vi "SwissSPAD Live_Decode SS3 FPGA Data_DVI.vi"(8 "Error In":errorcluster, 9 "Buffer Size (# 8-bit Images)":i32, 10 "SwissSPAD Live Internal Variables":T1={"okCFrontPanelDevices Refnum"=refnum, "Bottom Device Refnum"=refnum, "Display Image"=refnum, "# Live Images"=0, "relative s"=0.0, "# Image Sets"=0, "Message"="", "Current Image Set"=0, "# Datasets in Series"=0, "Current Dataset"=0, "Live Mode"=FALSE, "Recording Mode"=FALSE, "Record Button"=refnum, "\nLive Button"=refnum, "SwissSPAD Live Gate Image Data Q Name"="SS2 Live Gate Data Q", "Discard First Image"=FALSE, "Image Information"={"Save ROI Only"=FALSE, "Left"=0, "Top"=0, "Right"=0, "Bottom"=0, "Use Current ROI"=FALSE}, "Image Binning Options"={"Use Image Binning"=FALSE, "X Bin"=1, "Y Bin"=1}, "Bottom FPGA Serial Number"="", "Detector PCB Version"=enum."SS2 PCB1", "# Acquisitions"=1, "10 bits"=FALSE, "Top FPGA Serial Number"="", "Top Device Refnum"=refnum, "okCFrontPanel Refnum"=refnum} {"# Acquisitions" min=1; "Image Binning Options"."Y Bin" min=1; "Image Binning Options"."X Bin" min=1}) -> ()   [LabVIEW 2021]
uses:
  SwissSPAD Live_Internal Variables.ctl
  D:/UCLA Thinkpad Google Drive/LabVIEW 2021 SP1/builds/SwissSPAD Live Distribution/Opal Kelly/C# Wrapper/v5.0.2/libFrontPanel-csharp.dll
  Opal Kelly/C# Wrapper/v5.0.2/libFrontPanel-csharp.dll
  <vilib>/vision/Image Controls.llb/IMAQ Image.ctl
  SwissSPAD Live_Image ROI Information.ctl
  Phasor/Image Binning Options.ctl
  SwissSPAD Live_SSx PCB Version.ctl
  SwissSPAD Live_Settings List.ctl
  SwissSPAD Live_SS3 Displayed Image v2.ctl
  LV Tools/Logical Processors Used.vi
  Time/High Resolution Timing.vi
  <vilib>/vision/NI_Vision_Development_Module.lvlib
  Notebook/Notebook.lvlib
  Rich Text Box/Rich Text Box.lvlib
  Variant/Variant to Data/Variant to Data.lvlib
panel:
  out "# 8-bit image pairs queued":i32
  out "Activate Trigger Error Out":errorcluster
  out "8-bit Image Count":i32
  out "Error Out":errorcluster
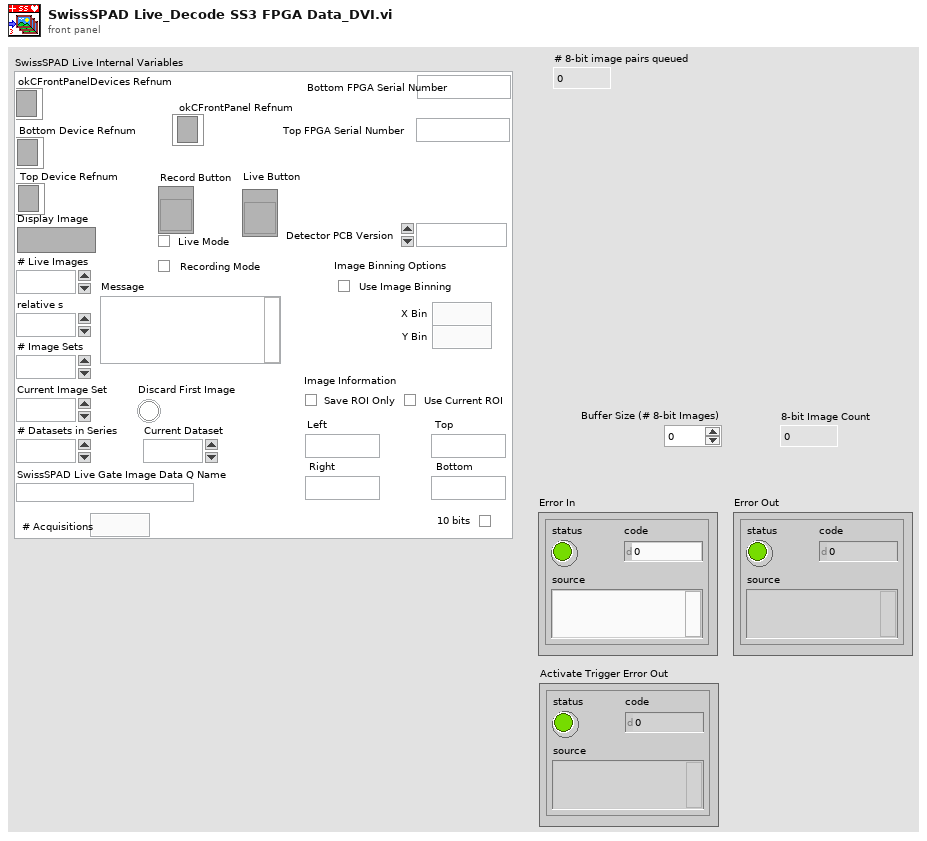
[diagram p1: front panel]
types:
  T1 = typedef "SwissSPAD Live_Internal Variables.ctl" = cluster{"okCFrontPanelDevices Refnum":refnum<k24>, "Bottom Device Refnum":refnum<k24>, "Display Image":T2, "# Live Images":i32, "relative s":dbl, "# Image Sets":i32, "Message":string, "Current Image Set":i32, "# Datasets in Series":i32, "Current Dataset":i32, "Live Mode":bool, "Recording Mode":bool, "Record Button":refnum<vi>, "\nLive Button":refnum<vi>, "SwissSPAD Live Gate Image Data Q Name":string, "Discard First Image":bool, "Image Information":T3, "Image Binning Options":T4, "Bottom FPGA Serial Number":string, "Detector PCB Version":T5, "# Acquisitions":u32, "10 bits":bool, "Top FPGA Serial Number":string, "Top Device Refnum":refnum<k24>, "okCFrontPanel Refnum":refnum<k24>}
  T2 = typedef "IMAQ Image.ctl" = refnum<image>
  T3 = typedef "SwissSPAD Live_Image ROI Information.ctl" = cluster{"Save ROI Only":bool, "Left":u16, "Top":u16, "Right":u16, "Bottom":u16, "Use Current ROI":bool}
  T4 = typedef "Image Binning Options.ctl" = cluster{"Use Image Binning":bool, "X Bin":i32, "Y Bin":i32}
  T5 = typedef "SwissSPAD Live_SSx PCB Version.ctl" = enum16{"unknown", "SS2 PCB1", "SS2 PCB2", "SS3 PCB1"}
  T6 = typedef "SwissSPAD Live_Settings List.ctl" = enum16{"FPGA:Bottom Half", "FPGA:Top Half", "FPGA:Bottom Bitfile Path", "FPGA:Top Bitfile Path", "FPGA:Bottom Bitstream Version", "FPGA:Top Bitstream Version", "FPGA:Auto Reset FPGA", "FPGA:Bottom FPGA Serial Number", "FPGA:Top FPGA Serial Number", "FPGA:Detector PCB Version", "Acquisition Parameters:Microlens", "Acquisition Parameters:SS2 DAQ Parameters", "Acquisition Parameters:Gate Configuration Array", "Acquisition Parameters:SS3 DAQ Parameters", "Acquisition Parameters:Buffer Size (# 8-bit Gates)", "File Information:File Information", "File Information:# Datasets in Series", "File Information:Scrambled File Flag", "File Information:SS3 Gate Slip Correction", "File Information:SS3 Hot Pixel Mismatch Detection", "File Information:Delay between Datasets", "File Information:Save Sum of All Gates Preview", "Image Parameters:Image ROI Information", "Image Parameters:Image Binning Options", "Image Parameters:SS3 Displayed Image", "Image Parameters:Image Display Options", "Image Parameters:Use Histogram Cursors", "Image Parameter:FPGA Data to Display", "UI Settings:Histogram Bins Number", "UI Settings:Histogram Bin Size", "UI Settings:Use Image Display Options", "UI Settings:Verbose Settings", "UI Settings:Verbose Saving"}
  T7 = typedef "SwissSPAD Live_SS3 Displayed Image v2.ctl" = enum16{"G2 Gate", "INT Gate", "INT - G2"}
  T8 = typedef "Image Type" = u32
  T9 = typedef "Rich Text Box.lvlib/Text Formatting.ctl" = cluster{"Font":string, "Text Color":T10, "Text Background Color":T10, "Text Style":enum16{"Regular", "Bold", "Italic", "Underline", "Strikeout"}, "Font Size (Points)":dbl, "Text Alignment":i32}
  T10 = typedef "Rich Text Box.lvlib/Text Colors.ctl" = enum16{"Unchanged", "Black", "Blue", "Brown", "Gray", "Green", "Orange", "Pink", "Red", "White"}
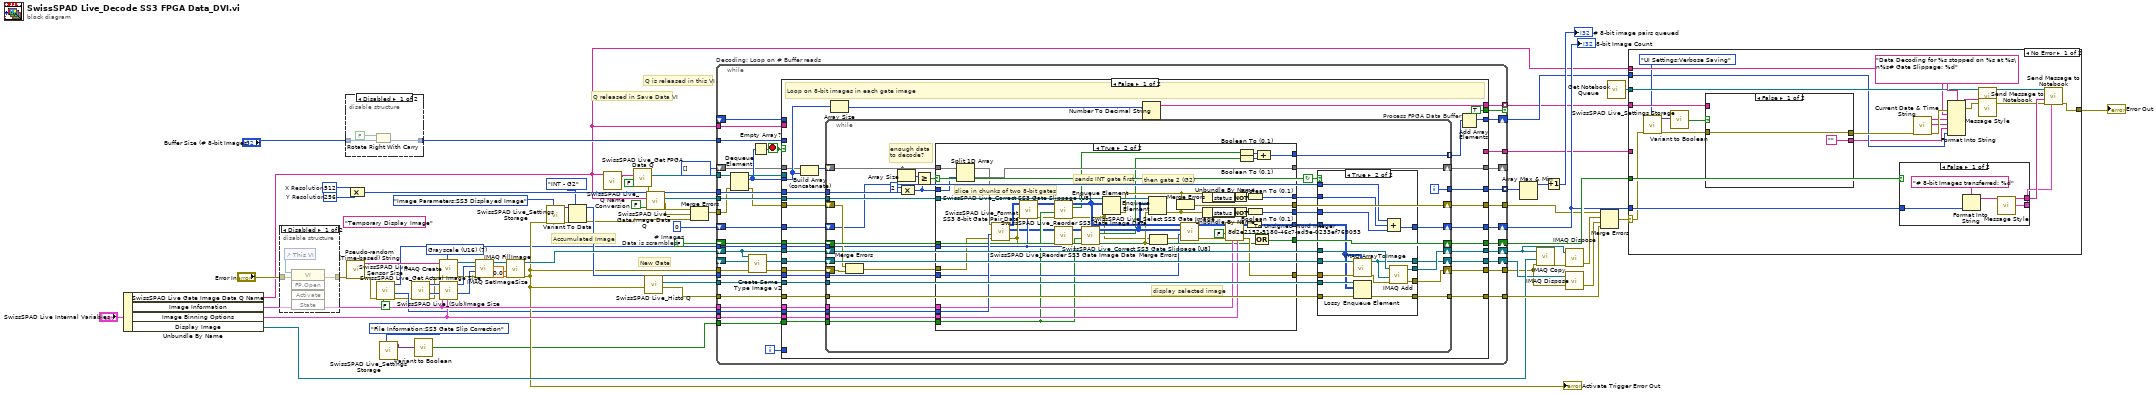
[diagram p0: block diagram]
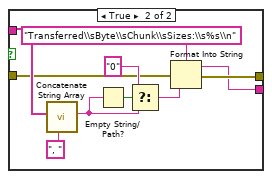
[diagram p3: hidden frame]
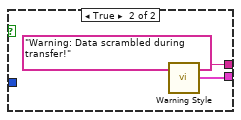
[diagram p4: hidden frame]
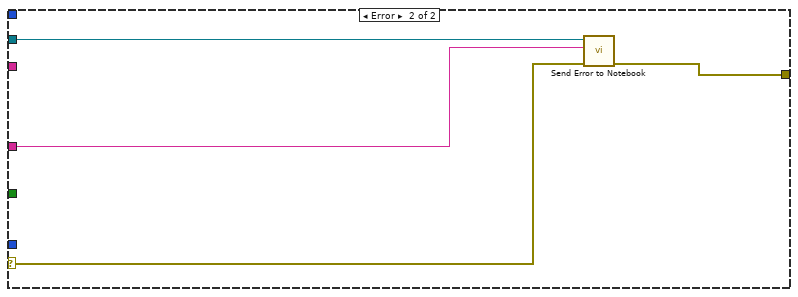
[diagram p5: hidden frame]
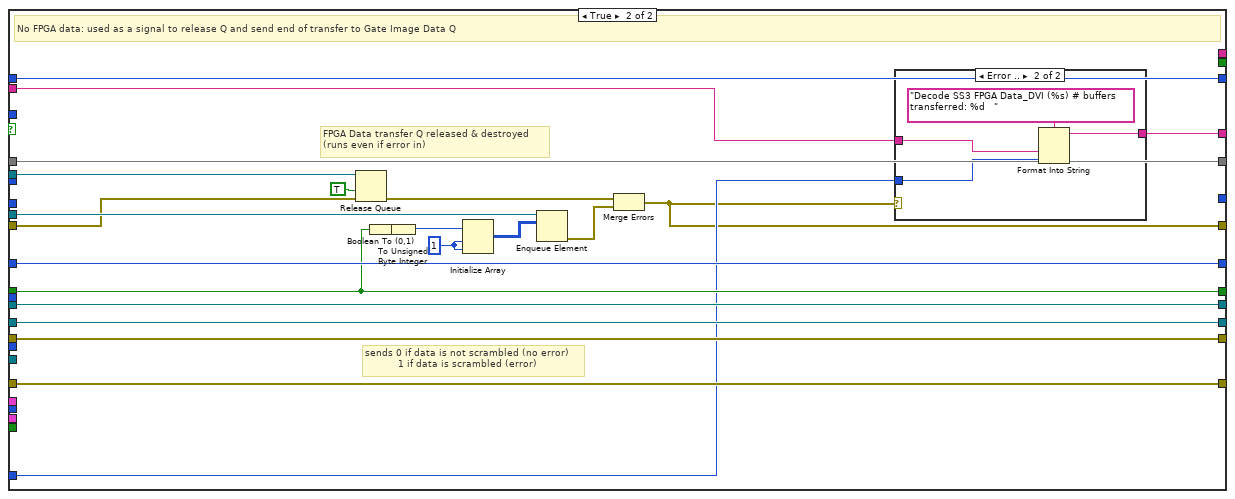
[diagram p8: hidden frame]
diagram:
  w56 = FALSE  # Data is scrambled
  w59 = T8 7 items=["Grayscale (U8)", "Grayscale (I16)", "Grayscale (SGL)", "Complex (CSG)", "RGB (U32)", "HSL (U32)", "RGB (U64)", "Grayscale (U16)"] ("Image Type")
  (unwired) "Temporary Display Image" ("Image Name")
  w68 = 0  # # Images
  w43 = 256  # Y Resolution
  w72 = 512  # X Resolution
  # "New Gate"
  # "Accumulated Image"
  # "Q released in Save Data VI"
  # "Q is released in this VI"
  n1 = Unbundle By Name("SwissSPAD Live Internal Variables") -> ("SwissSPAD Live Gate Image Data Q Name"=w8:string, "Image Information"=w55:T3, "Image Binning Options"=w54:T4, "Display Image"=w52:T2)
  n2 = disable-structure shown="Disabled" {
    disable-tunnel: "Error In" -> [w74 w76]
    disable-tunnel: [w73 w76] -> w35
    frame Disabled {
      n3 = control-ref of="This VI"() -> (w75:refnum<vi>)
      n4 = invoke class="VI" method="FP.Open"(reference=w75, error in=w74) -> (error out=w73:errorcluster)  [unwired: 3 in, 4 out]
    }
    frame Enabled {
    }
  }
  n5 = disable-structure shown="Disabled" {
    disable-tunnel: [w79 w80] -> w39
    disable-tunnel: "Buffer Size (# 8-bit Images)" -> [w78 w80]
    frame Disabled {
      n6 = Rotate Right With Carry(2:w78, 3:FALSE ("carry")) -> (0:w79:i32)  [unwired: 1 out]
    }
    frame Enabled {
      # "Divide by 2 to obtain # INT+G2 pairs"
    }
  }
  n7 = call "Pseudo-random (Time-based) String.vi"("Error In"=w35) -> ("Error Out"=w10:errorcluster, "result string"=w47:string)  [unwired: 9 in]
  n8 = Compound Arithmetic op=MULTIPLY(w72, w43) -> (w58:i32)
  n9 = call "SwissSPAD Live_Sensor Size.vi"("Set/Get(F)"=FALSE, "Error In"=w10) -> ("Error Out"=w14:errorcluster, "Y size"=w16:i32, "X size"=w17:i32)  [unwired: 7 in]
  n10 = call "SwissSPAD Live_Settings Storage.vi"("Settings List"=SwissSPAD_Live_Settings_List."File Information:SS3 Gate Slip Correction") -> ("Variant Data out"=w4:variant)  [unwired: 9 in, 1 out]
  n11 = call "SwissSPAD Live_Get Actual Image Size.vi"("error in (no error)"=w14) -> ("error out"=w11:errorcluster, "Y size"=w12:i32, "X size"=w13:i32)  [unwired: 8 in]
  n12 = call "Variant to Boolean.vi"("Variant"=w4) -> ("Value"=w18:bool)  [unwired: 8 in]
  n13 = call "IMAQ Create"("Image Name"=w47, "Image Type"=w59, "error in (no error)"=w11) -> ("New Image"=w64:T2, "error out"=w65:errorcluster)  [unwired: 2 in]
  n14 = call "SwissSPAD Live_(Sub)Image Size.vi"("Image Binning Options"=w54, "Image Information"=w55, "# Pixel Y in"=w12, "# Pixel X in"=w13) -> ("# Pixel Y out"=w66:i32, "# Pixel X out"=w67:i32)  [unwired: 6 in]
  n15 = call "IMAQ SetImageSize"("error in (no error)"=w65, "Y Resolution"=w66, "X Resolution"=w67, "Image"=w64) -> ("error out"=w62:errorcluster, "Image Out"=w63:T2)  [unwired: 1 in]
  n16 = call "IMAQ FillImage"("error in (no error)"=w62, "Pixel Value (U8, U16, I16, Float)"=sgl 0.0, "Image"=w63) -> ("error out"=w19:errorcluster, "Image Out"=w61:T2)  [unwired: 7 in]
  "Activate Trigger Error Out" <- w19
  n17 = call "SwissSPAD Live_Settings Storage.vi"("Settings List"=SwissSPAD_Live_Settings_List."Image Parameters:SS3 Displayed Image", "Error In"=w19) -> ("Error Out"=w46:errorcluster, "Variant Data out"=w3:variant)  [unwired: 8 in]
  n18 = Variant To Data(error in=w46, type=SwissSPAD_Live_SS3_Displayed_Image_v2."INT - G2" ("Image to Display"), Variant=w3) -> (data=w44:T7, error out=w7:errorcluster)
  n19 = call "SwissSPAD Live_Q Name Conversion.vi"("SwissSPAD Live Gate Data Decode Q Name"=w8) -> ("FPGA Q Name"=w28:string)  [unwired: 10 in]
  n20 = call "SwissSPAD Live_Get FPGA Data Q.vi"("create if not found? (T)"=FALSE, "FPGA Data Q Name"=w28) -> ("error out"=w22:errorcluster, "FPGA Data Q"=w32:refnum<queue>)  [unwired: 8 in]
  n21 = call "SwissSPAD Live_Histo Q.vi"("error in (no error)"=w19) -> ("error out"=w70:errorcluster, "SS2 Live Histo Q"=w71:refnum<queue>)  [unwired: 5 in]
  n22 = call "SwissSPAD Live_Gate Image Data Q.vi"("create if not found? (T)"=FALSE, "SwissSPAD Live Gate Image Data Q Name"=w8) -> ("error out"=w21:errorcluster, "SwissSPAD Live Gate Image Data Q"=w31:refnum<queue>)  [unwired: 7 in, 1 out]
  n23 = Merge Errors(w22, w21, w7) -> (w23:errorcluster)
  n24 = while "Decoding: Loop on # Buffer reads" {
    tunnel: w16 -> [w121]
    tunnel: w19 -> [w114]
    tunnel: w39 -> [w120]
    tunnel: w58 -> [w119]
    shift-right: [w105] -> w26
    shift-left: _ -> [w117]
    tunnel: [w118] -> w25
    tunnel: w23 -> [w103]
    tunnel: [w111] -> w34
    tunnel: w71 -> [w110]
    tunnel: w70 -> [w109]
    tunnel: [w108] -> w69
    shift-right: [w107] -> w50
    shift-left: w61 -> [w116]
    tunnel: w32 -> [w104]
    shift-right: [w113] -> w37
    shift-left: w68 -> [w100]
    tunnel: w55 -> [w99]
    tunnel: w54 -> [w98]
    shift-right: [w97] -> w57
    shift-left: w56 -> [w96]
    tunnel: w17 -> [w94]
    tunnel: w44 -> [w93]
    tunnel: [w92] -> w42 mode=indexing
    tunnel: w31 -> [w112]
    tunnel: [w90] -> w27
    tunnel: w8 -> [w89]
    tunnel: [w88] -> w1 mode=indexing if=w83
    tunnel: w18 -> [w87]
    shift-right: [w85] -> w9
    shift-left: _ -> [w84]
    shift-right: [w81] -> _
    shift-left: u8[] [] -> [w82]
    i -> [w91]
    stop <- w101 stop-if-true
    n25 = Dequeue Element(queue=w104, error in (no error)=w103) -> (queue out=w95:refnum<queue>, element=w86:u8[], error out=w102:errorcluster)  [unwired: 1 in, 1 out]
    n26 = call "Create Same Type Image v2.vi"("error in (no error)"=w114, "Image Dst"=w117, "Image Src"=w116) -> ("error out"=w115:errorcluster, "Image Dst"=w106:T2)  [unwired: 6 in, 1 out]
    n27 = Empty Array?(array=w86) -> (empty?=w101:bool)
    n28 = case shown="False" w101 {
      tunnel: w121 -> [w154 _]
      tunnel: w120 -> [_ _]
      tunnel: w119 -> [w153 _]
      tunnel: [w152 w280] -> w118
      tunnel: w116 -> [w151 w282]
      tunnel: w115 -> [w150 w280]
      tunnel: [w138 w283] -> w113
      tunnel: w112 -> [w149 w278]
      tunnel: [w148 w267] -> w111
      tunnel: w110 -> [w147 _]
      tunnel: w109 -> [w146 w279]
      tunnel: [w145 w279] -> w108
      tunnel: [w144 w282] -> w107
      tunnel: w106 -> [w143 w281]
      tunnel: [w142 w281] -> w105
      tunnel: w102 -> [w141 w268]
      tunnel: w86 -> [w131 _]
      tunnel: w100 -> [w139 w283]
      tunnel: w99 -> [w140 _]
      tunnel: w98 -> [w137 _]
      tunnel: [w135 w277] -> w97
      tunnel: w96 -> [w136 w277]
      tunnel: w95 -> [_ w272]
      tunnel: w94 -> [w134 _]
      tunnel: w93 -> [w133 _]
      tunnel: [w132 _] -> w92
      tunnel: w91 -> [_ w270]
      tunnel: [_ w265] -> w90
      tunnel: w89 -> [_ w264]
      tunnel: [w129 _] -> w88
      tunnel: w87 -> [w128 _]
      tunnel: [w126 w263] -> w85
      tunnel: w84 -> [_ w263]
      tunnel: [TRUE _] -> w83
      tunnel: w82 -> [w123 w262]
      tunnel: [w122 w262] -> w81
      frame False {
        # "Loop on 8-bit images in each gate image"
        n29 = Build Array (concatenate)(w123, w131) -> (w124:u8[])
        n30 = while "Process FPGA Data Buffer" {
          tunnel: w154 -> [w190]
          shift-right: [w184] -> w152
          shift-left: w150 -> [w189]
          shift-right: [w183] -> w122
          shift-left: w124 -> [w188]
          tunnel: w153 -> [w187]
          shift-right: [w165] -> w148
          shift-left: w141 -> [w170]
          tunnel: w147 -> [w182]
          tunnel: w146 -> [w181]
          tunnel: [w180] -> w145
          shift-right: [w179] -> w144
          shift-left: w151 -> [w185]
          shift-right: [w178] -> w142
          shift-left: w143 -> [w186]
          tunnel: w140 -> [w175]
          shift-right: [w176] -> w138
          shift-left: w139 -> [w159]
          tunnel: w137 -> [w174]
          shift-right: [w172] -> w135
          shift-left: w136 -> [w173]
          tunnel: w134 -> [w167]
          tunnel: w133 -> [w166]
          tunnel: [w169] -> w132
          tunnel: w149 -> [w171]
          tunnel: w128 -> [w162]
          tunnel: [w161] -> w127 mode=indexing
          i -> [w169]
          stop <- w158 continue-if-true
          # "enough data to decode?"
          n31 = Merge Errors(w170, w189) -> (w160:errorcluster)
          n32 = Array Size(array=w188) -> (size(s)=w156:i32)
          n33 = Compound Arithmetic op=MULTIPLY(2 ("value"), w187) -> (w155:i32)
          n34 = Greater Or Equal?(x=w156, y=w155) -> (x >= y?=w158:bool)
          n35 = case shown="True" w158 {
            tunnel: w190 -> [_ w241]
            tunnel: [w193 w240] -> w183
            tunnel: [w192 w239] -> w177
            tunnel: w175 -> [_ w238]
            tunnel: w174 -> [_ w237]
            tunnel: w173 -> [w191 w236]
            tunnel: [w191 w235] -> w172
            tunnel: w171 -> [_ w234]
            tunnel: [_ w233] -> w168
            tunnel: w167 -> [_ w232]
            tunnel: w166 -> [_ w231]
            tunnel: [w192 w230] -> w165
            tunnel: [_ w229] -> w164
            tunnel: [_ w228] -> w163
            tunnel: w162 -> [_ w227]
            tunnel: [_ w226] -> w161
            tunnel: w160 -> [w192 w220]
            tunnel: w188 -> [w193 w195]
            tunnel: w155 -> [_ w194]
            frame False {
            }
            frame True {
              # "slice in chunks of two 8-bit gates"
              # "display selected image"
              # "then gate 2 (G2)"
              # "sends INT gate first"
              n36 = Split 1D Array(array=w195, index=w194) -> (first subarray=w225:u8[], second subarray=w240:u8[])
              n37 = call "SwissSPAD Live_Format SS3 8-bit Gate Pair Data.vi"("Error In"=w220, "Y Resolution (250)"=w241, "Flattened Image (512x256x2)"=w225) -> ("Error Out"=w219:errorcluster, "Gate 2 (512x250)"=w210:u8[][], "Integral Gate (512x250)"=w209:u8[][])  [unwired: 6 in]
              n38 = call "SwissSPAD Live_Reorder SS3 Gate Image Data.vi"("X Resolution (500)"=w232, "Error In"=w219, "Interlaced Gate (512x250)"=w209) -> ("Error Out"=w207:errorcluster, "De-interlaced Gate (500x250)"=w208:u8[][])  [unwired: 7 in]
              n39 = call "SwissSPAD Live_Correct SS3 Gate Slippage [U8].vi"("Error In"=w207, "Slippage Correction (T)"=w227, "Array in"=w208) -> ("Error Out"=w197:errorcluster, "Last Strip Saturated?"=w202:bool, "Array out"=w206:u8[][])  [unwired: 6 in]
              n40 = call "SwissSPAD Live_Reorder SS3 Gate Image Data.vi"("X Resolution (500)"=w232, "Error In"=w219, "Interlaced Gate (512x250)"=w210) -> ("Error Out"=w204:errorcluster, "De-interlaced Gate (500x250)"=w205:u8[][])  [unwired: 7 in]
              n41 = call "SwissSPAD Live_Correct SS3 Gate Slippage [U8].vi"("Error In"=w204, "Slippage Correction (T)"=w227, "Array in"=w205) -> ("Error Out"=w198:errorcluster, "Last Strip Saturated?"=w200:bool, "Array out"=w203:u8[][])  [unwired: 6 in]
              n42 = Enqueue Element(queue=w234, element=w206, error in (no error)=w197) -> (queue out=w221:refnum<queue>, error out=w216:errorcluster)  [unwired: 1 in, 1 out]
              n43 = Enqueue Element(queue=w221, element=w203, error in (no error)=w198) -> (error out=w211:errorcluster)  [unwired: 1 in, 2 out]
              n44 = Merge Errors(w197, w198) -> (w217:errorcluster)
              n45 = Merge Errors(w216, w211) -> (w230:errorcluster)
              n46 = call "SwissSPAD Live_Select SS3 Gate Image.vi"("Error In"=w217, "Image to Display"=w231, "Gate 2 (500x250)"=w203, "INT Gate (500x250)"=w206) -> ("Error Out"=w218:errorcluster, "Selected Gate (500x250)"=w222:u8[][])  [unwired: 5 in, 1 out]
              n47 = Unbundle By Name(w216) -> ("status"=w215:bool)
              n48 = Unbundle By Name(w211) -> ("status"=w212:bool)
              n49 = call "8d2e2152-5180-46c7-ad9e-0233ef769053.vi"("Image Binning Options"=w237, "Image Information"=w238, "Error In"=w218, "Test for scrambling"=FALSE, "Image in"=w222) -> ("Error Out"=w239:errorcluster, "Data is scrambled"=w223:bool, "Image out"=w224:u8[][])  [unwired: 4 in]
              n50 = Not(x=w215) -> (.not. x?=w214:bool)
              n51 = Not(x=w212) -> (.not. x?=w213:bool)
              n52 = Boolean To (0,1)(Boolean=w202) -> (0, 1=w201:i16)
              n53 = Boolean To (0,1)(Boolean=w200) -> (0, 1=w199:i16)
              n54 = To Unsigned Word Integer(number=w224) -> (unsigned 16bit integer=w233:u16[][])
              n55 = Boolean To (0,1)(Boolean=w214) -> (0, 1=w229:i16)
              n56 = Boolean To (0,1)(Boolean=w213) -> (0, 1=w228:i16)
              n57 = Compound Arithmetic op=OR(w223, w236) -> (w235:bool)
              n58 = Compound Arithmetic op=ADD(w201, w199) -> (w226:i16)
            }
          }
          n59 = case shown="True" w158 {
            tunnel: w186 -> [w244 w261]
            tunnel: w185 -> [w243 w260]
            tunnel: [w245 w259] -> w184
            tunnel: w182 -> [_ w258]
            tunnel: w181 -> [w246 w257]
            tunnel: [w246 w256] -> w180
            tunnel: [w243 w255] -> w179
            tunnel: [w244 w254] -> w178
            tunnel: w177 -> [w245 w253]
            tunnel: [w242 w252] -> w176
            tunnel: w168 -> [_ w251]
            tunnel: w164 -> [_ w250]
            tunnel: w163 -> [_ w249]
            tunnel: w159 -> [w242 w248]
            frame False {
            }
            frame True {
              n60 = call "IMAQ ArrayToImage"("Image Pixels (U16)"=w251, "error in (no error)"=w253, "Image"=w261) -> ("error out"=w247:errorcluster, "Image Out"=w254:T2)  [unwired: 7 in]
              n61 = Lossy Enqueue Element(queue=w258, element=w251, error in (no error)=w257) -> (error out=w256:errorcluster)  [unwired: 3 out]
              n62 = Compound Arithmetic op=ADD(w248, w250, w249) -> (w252:i32)
              n63 = call "IMAQ Add"("Image Src A"=w260, "Image Src B"=w254, "error in (no error)"=w247) -> ("Image Dst Out"=w255:T2, "error out"=w259:errorcluster)  [unwired: 4 in]
            }
          }
        }
        n64 = Array Size(array=w131) -> (size(s)=w130:i32)
        n65 = Number To Decimal String(number=w130) -> (decimal integer string=w129:string)  [unwired: 1 in]
        n66 = Add Array Elements(numeric array=w127) -> (sum=w126:i16)
      }
      frame True {
        w274 = 1 ("dimension size")
        # "FPGA Data transfer Q released & destroyed\n(runs even if error in)"
        # "sends 0 if data is not scrambled (no error)\n           1 if data is scrambled (error)"
        # "No FPGA data: used as a signal to release Q and send end of transfer to Gate Image Data Q"
        n67 = Release Queue(queue=w272, force destroy? (F)=TRUE, error in (no error)=w268) -> (error out=w266:errorcluster)  [unwired: 2 out]
        n68 = Boolean To (0,1)(Boolean=w277) -> (0, 1=w276:i16)
        n69 = To Unsigned Byte Integer(number=w276) -> (unsigned 8bit integer=w275:u8)
        n70 = Initialize Array(w275, w274, w274) -> (w273:u8[][])
        n71 = Enqueue Element(queue=w278, element=w273) -> (error out=w271:errorcluster)  [unwired: 2 in, 2 out]
        n72 = Merge Errors(w266, w271) -> (w267:errorcluster)
        n73 = case shown="Error .." w267 {
          tunnel: w270 -> [_ w285]
          tunnel: [_ w286] -> w265
          tunnel: w264 -> [_ w284]
          frame No Error {
          }
          frame Error {
            n74 = Format Into String(format string="Decode SS3 FPGA Data_DVI (%s) # buffers transferred: %d   ", w284, w285) -> (resulting string=w286:string)  [unwired: 2 in, 1 out]
          }
        }
      }
    }
  }
  "8-bit Image Count" <- w37
  n75 = Array Max & Min(array=w42) -> (max value=w41:i32)  [unwired: 3 out]
  n76 = call "IMAQ Copy"("error in (no error)"=w25, "Image Dst"=w52, "Image Src"=w50) -> ("error out"=w49:errorcluster)  [unwired: 3 in, 1 out]
  n77 = Increment(x=w41) -> (x+1=→"# 8-bit image pairs queued":i32)
  n78 = call "IMAQ Dispose"("Image"=w50, "error in (no error)"=w49) -> ("error out"=w48:errorcluster)  [unwired: 4 in]
  n79 = call "IMAQ Dispose"("Image"=w26, "error in (no error)"=w25) -> ("error out"=w24:errorcluster)  [unwired: 4 in]
  n80 = Merge Errors(w34, w48, w24, w69) -> (w33:errorcluster)
  n81 = call "Get Notebook Queue.vi"() -> ("Notebook Queue"=w36:refnum<queue>)  [unwired: 9 in]
  n82 = case shown="No Error" w33 {
    selector: w33 -> [w293 w333]
    tunnel: w57 -> [w312 _]
    tunnel: w37 -> [w305 _]
    tunnel: w36 -> [w301 w334]
    tunnel: w27 -> [_ w332]
    tunnel: [w300 w331] -> w20
    tunnel: w9 -> [w291 _]
    tunnel: w8 -> [w298 _]
    tunnel: w1 -> [w296 _]
    frame No Error {
      n83 = call "SwissSPAD Live_Settings Storage.vi"("Settings List"=SwissSPAD_Live_Settings_List."UI Settings:Verbose Saving", "Error In"=w293) -> ("Error Out"=w294:errorcluster, "Variant Data out"=w289:variant)  [unwired: 8 in]
      n84 = call "Variant to Boolean.vi"("Variant"=w289) -> ("Value"=w288:bool)  [unwired: 8 in]
      n85 = case shown="False" w288 {
        tunnel: w296 -> [_ w321]
        tunnel: w294 -> [w314 w317]
        tunnel: [w314 w316] -> w292
        tunnel: ["" w315] -> w290
        frame False {
        }
        frame True {
          n86 = call "Concatenate String Array.vi"("Separator (TAB)"=", ", "String Array"=w321) -> ("Formatted String"=w320:string)  [unwired: 9 in]
          n87 = Empty String/Path?(string/path=w320) -> (empty?=w324:bool)
          n88 = Select(t="0" ("Formatted String"), s=w324, f=w320) -> (s? t:f=w319:string)
          n89 = Format Into String(format string="Transferred\\sByte\\sChunk\\sSizes:\\s%s\\n", error in=w317, w319) -> (resulting string=w315:string, error out=w316:errorcluster)  [unwired: 1 in]
        }
      }
      n90 = case shown="False" w312 {
        tunnel: w305 -> [w328 _]
        tunnel: [w325 "Warning: Data scrambled during transfer!" ("format string")] -> w304
        tunnel: [w326 w329] -> w303
        frame False {
          n91 = Format Into String(format string="# 8-bit Images transferred: %d", w328) -> (resulting string=w325:string)  [unwired: 2 in, 1 out]
          n92 = call "Message Style.vi"() -> ("Message Formatting"=w326:T9)
        }
        frame True {
          n93 = call "Warning Style.vi"() -> ("Error Formatting"=w329:T9)
        }
      }
      n94 = call "Current Date & Time String.vi"("Error In"=w292) -> ("Error Out"=w308:errorcluster, "time string"=w306:string, "date string"=w299:string)  [unwired: 8 in]
      n95 = Format Into String(format string="Data Decoding for %s stopped on %s at %s\n%s# Gate Slippage: %d", error in=w308, w298, w299, w306, w290, w291) -> (resulting string=w310:string, error out=w307:errorcluster)  [unwired: 1 in]
      n96 = call "Message Style.vi"() -> ("Message Formatting"=w309:T9)
      n97 = call "Send Message to Notebook.vi"("Text Formatting"=w309, "Error In"=w307, "Message"=w310, "Notebook Queue"=w301) -> ("Error Out"=w302:errorcluster, "Notebook Queue"=w297:refnum<queue>)  [unwired: 4 in]
      n98 = call "Send Message to Notebook.vi"("Text Formatting"=w303, "Error In"=w302, "Message"=w304, "Notebook Queue"=w297) -> ("Error Out"=w300:errorcluster)  [unwired: 4 in, 1 out]
    }
    frame Error {
      n99 = call "Send Error to Notebook.vi"("error in (no error)"=w333, "State Machine Case Error Source"=w332, "Notebook Q"=w334) -> ("Error Out"=w331:errorcluster)  [unwired: 8 in]
    }
  }
  "Error Out" <- w20
